vi "Read from Fixture Config.vi"(9 "error in (no error)":errorcluster, 10 "Key":string, 11 "Test Class in":refnum<class "Test Class.lvclass">) -> (1 "error out":errorcluster, 3 "Instrument Info":string)   [LabVIEW 2017, in "Test Class.lvclass"]
uses:
  Test Class.lvclass
  Classes/Station Config/Fixture Config/Fixture Config.lvclass
  C:/Test System Services/Acrobat Framework/CBTF Modules/Classes/Station Config/Class/Station Config.lvclass
  Classes/Station Config/Class/Station Config.lvclass
  Classes/Test Recipe/Class/Test Recipe.lvclass
  Classes/Application/Class/Application.lvclass
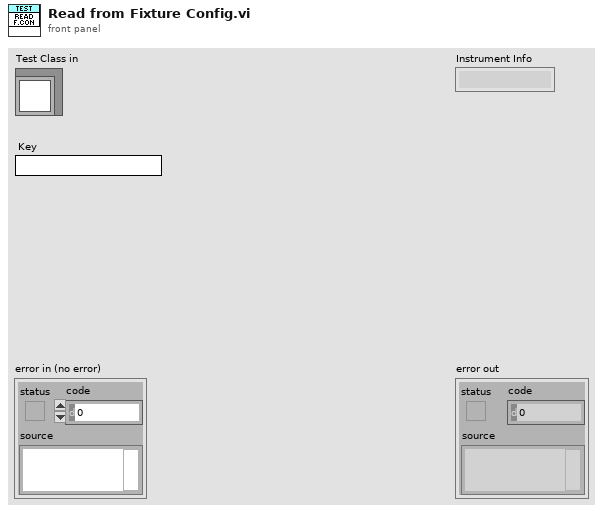
[diagram p1: front panel]
types:
  T1 = typedef "Application.lvlib/App Properties.lvclass/Class Properties -- Cluster.ctl" = cluster{"UUT Info":T2[], "Test Information":refnum<vi>, "Gold Board":refnum<class "Golden Board.lvclass">, "Test Recipe":refnum<class "Test Recipe.lvclass">, "Instruments":refnum<class "Instrument.lvclass">[], "Mode":T3, "Test Results":T4[], "Station Config":refnum<class "Station Config.lvclass">, "Variable Engine":refnum<class "Variable Engine.lvclass">}
  T2 = typedef "Application.lvlib/App Properties.lvclass/UUT Reference -- Cluster.ctl" = cluster{"Serial Number Reference":refnum<vi>, "Status Message Reference":refnum<vi>}
  T3 = typedef "Application.lvlib/Application.lvclass/Op Mode -- Enum.ctl" = u16
  T4 = typedef "Application.lvlib/App Properties.lvclass/Test Result -- Cluster.ctl" = cluster{"Position":i32, "Pass":bool, "Fail Codes":string}
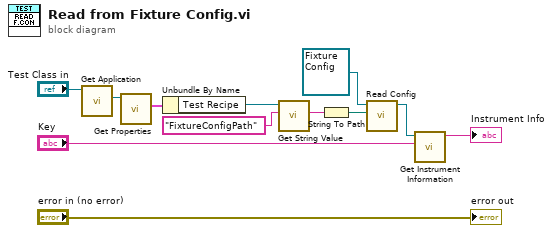
[diagram p0: block diagram]
diagram:
  n1 = call "Get Application.vi"("Test Class in"="Test Class in") -> ("Application.lvlib:Application.lvclass"=w3:refnum<class "Application.lvclass">)  [unwired: 9 in, 1 out]
  n2 = call "Get Properties.vi"("Acrobat Template in"=w3) -> ("Class Properties"=w10:T1)  [unwired: 8 in, 2 out]
  n3 = Unbundle By Name(w10) -> ("Test Recipe"=w9:refnum<class "Test Recipe.lvclass">)
  n4 = call "Get String Value.vi"("Name"="FixtureConfigPath", "Test Recipe in"=w9) -> ("Value"=w7:string)  [unwired: 6 in, 3 out]
  n5 = String To Path(string=w7) -> (path=w6:path)
  n6 = call-dynamic "Read Config.vi"("Path to Config Folder"=w6, "Fixture Config in"=refnum<class "Fixture Config.lvclass"> refnum ("Station Config.lvlib:Fixture Config.lvclass")) -> ("Fixture Config out"=w5:refnum<class "Fixture Config.lvclass">)  [unwired: 8 in, 1 out]
  n7 = call "Get Instrument Information.vi"("Information Tag"="Key", "Station Config in"=w5) -> ("Instrument Info"=→"Instrument Info":string)  [unwired: 8 in, 1 out]
  "error out" <- "error in (no error)"
